vi "CheckStatus_Power_HeaterAlarm.vi"(8 "error in (no error)":errorcluster, 10 "RelayKeyStatus":bool, 11 "DAQmxTaksContainer_General in":refnum<class "DAQmxTaksContainer_General.lvclass">) -> (0 "error out":errorcluster, 1 "PowerStatus":bool, 2 "PowerStatusChanged":bool, 3 "DAQmxTaksContainer_General out":refnum<class "DAQmxTaksContainer_General.lvclass">, 4 "DAQmxTaskAICurrent en sortie":refnum<class "DAQmxTaskAICurrent_General.lvclass">, 5 "HeaterAlarmStatus":bool, 7 "HeaterAlarmStatusChanged":bool)   [LabVIEW 2018, in "DAQmxTaksContainer_General.lvclass"]
uses:
  DAQmxTaksContainer_General.lvclass
  DAQmxTaskAICurrent_General/DAQmxTaskAICurrent_General.lvclass
  DAQmxTaksContainer_General.lvclass/DAQmxTaksContainer_General.ctl
  DAQmxTaskAICurrent_General/DAQmxTaskAICurrent_General.lvclass/DAQmxTaskAICurrent_General.ctl
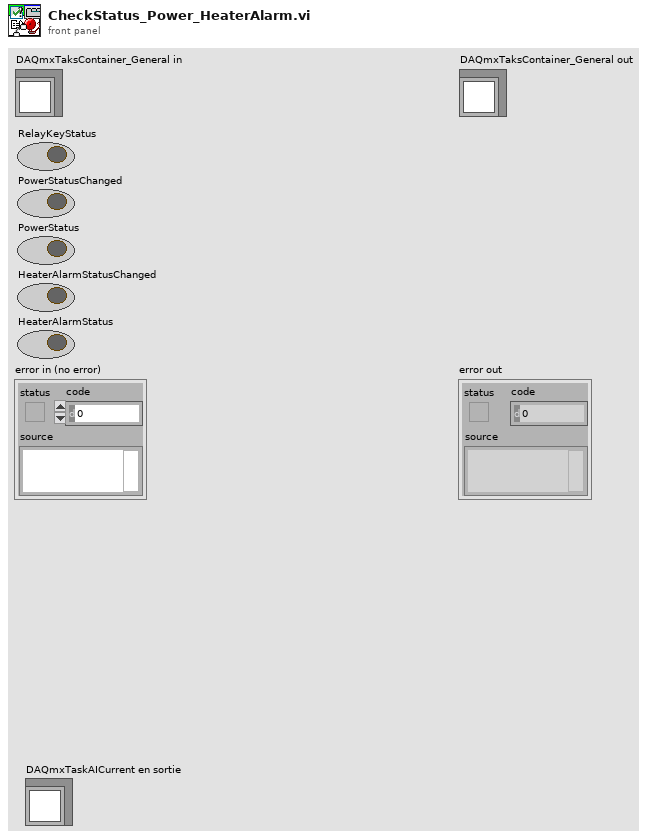
[diagram p1: front panel]
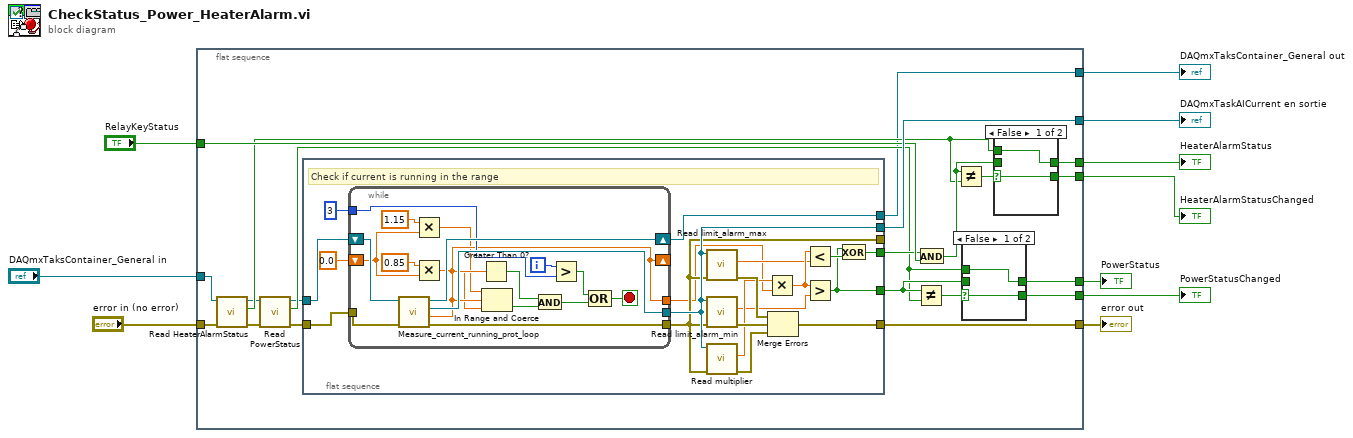
[diagram p0: block diagram]
diagram:
  n1 = flat-sequence {
    tunnel: "DAQmxTaksContainer_General in" -> [w17]
    tunnel: "error in (no error)" -> [w15]
    tunnel: [w31] -> w1
    tunnel: [w30] -> w5
    tunnel: "RelayKeyStatus" -> [w29]
    tunnel: [w25] -> w7
    tunnel: [w24] -> w8
    tunnel: [w22] -> w9
    tunnel: [w20] -> w10
    tunnel: [w11] -> w2
    frame #0 {
      n2 = call "Read HeaterAlarmStatus.vi"("error in (no error)"=w15, "DAQmxTaksContainer_General in"=w17) -> ("error out"=w14:errorcluster, "HeaterAlarmStatus"=w19:bool, "DAQmxTaksContainer_General out"=w16:refnum<class "DAQmxTaksContainer_General.lvclass">)  [unwired: 7 in]
      n3 = call "Read PowerStatus.vi"("error in (no error)"=w14, "DAQmxTaksContainer_General in"=w16) -> ("error out"=w13:errorcluster, "PowerStatus"=w18:bool, "DAQmxTaksContainer_General out"=w12:refnum<class "DAQmxTaksContainer_General.lvclass">)  [unwired: 7 in]
      n4 = flat-sequence {
        tunnel: [w44] -> w31
        tunnel: [w43] -> w30
        tunnel: [w42] -> _
        tunnel: [w39] -> w28
        tunnel: [w38] -> w26
        tunnel: w13 -> [w37]
        tunnel: w12 -> [w36]
        tunnel: [w35] -> w11
        frame #0 {
          # "Check if current is running in the range"
          n5 = while {
            tunnel: [w68] -> w43
            tunnel: [w56] -> w34
            shift-right: [w64] -> w35
            shift-left: w36 -> [w65]
            tunnel: w37 -> [w66]
            tunnel: [w67] -> w42
            shift-right: [w56] -> _
            shift-left: 0.0 ("value") -> [w53]
            tunnel: 3 -> [w62]
            i -> [w63]
            stop <- w60 stop-if-true
            n6 = call "Measure_current_running_prot_loop.vi"("error in (no error)"=w66, "DAQmxTaksContainer_General in"=w65) -> ("error out"=w67:errorcluster, "value"=w56:dbl, "DAQmxTask en sortie"=w68:refnum<class "DAQmxTaskAICurrent_General.lvclass">, "DAQmxTaksContainer_General out"=w64:refnum<class "DAQmxTaksContainer_General.lvclass">)  [unwired: 6 in]
            n7 = Multiply(x=1.15, y=w53) -> (x*y=w55:dbl)
            n8 = Multiply(x=0.85, y=w53) -> (x*y=w54:dbl)
            n9 = Greater Than 0?(x=w56) -> (x > 0?=w59:bool)
            n10 = In Range and Coerce(upper limit=w55, x=w56, lower limit=w54) -> (In Range?=w57:bool)  [unwired: 1 out]
            n11 = And(x=w59, y=w57) -> (x .and. y?=w58:bool)
            n12 = Greater?(x=w63, y=w62) -> (0:w61:bool)
            n13 = Compound Arithmetic op=OR(w61, w58) -> (w60:bool)
          }
          n14 = call "Read limit_alarm_max.vi"("error in (no error)"=w42, "DAQmxTaskAICurrent_General in"=w43) -> ("error out"=w46:errorcluster, "limit_alarm_max"=w40:dbl)  [unwired: 7 in, 1 out]
          n15 = call "Read limit_alarm_min.vi"("error in (no error)"=w42, "DAQmxTaskAICurrent_General in"=w43) -> ("error out"=w47:errorcluster, "limit_alarm_min"=w41:dbl)  [unwired: 7 in, 1 out]
          n16 = call "Read multiplier.vi"("error in (no error)"=w42, "DAQmxTaskAICurrent_General in"=w43) -> ("error out"=w48:errorcluster, "multiplier"=w45:dbl)  [unwired: 7 in, 1 out]
          n17 = Multiply(x=w45, y=w34) -> (x*y=w49:dbl)
          n18 = Merge Errors(w46, w47, w48) -> (w44:errorcluster)
          n19 = Less?(x=w49, y=w40) -> (x < y?=w50:bool)
          n20 = Greater?(x=w49, y=w41) -> (0:w38:bool)
          n21 = Exclusive Or(1:w50, 2:w38) -> (0:w39:bool)
        }
      }
      n22 = Not Equal?(x=w26, y=w18) -> (x != y?=w27:bool)
      n23 = And(x=w28, y=w29) -> (x .and. y?=w21:bool)
      n24 = Not Equal?(x=w21, y=w19) -> (x != y?=w23:bool)
      n25 = case shown="False" w27 {
        selector: w27 -> [w74 w75]
        tunnel: [w74 w75] -> w25
        tunnel: w26 -> [_ w76]
        tunnel: [w73 w76] -> w24
        tunnel: w18 -> [w73 _]
        frame False {
        }
        frame True {
        }
      }
      n26 = case shown="False" w23 {
        selector: w23 -> [w70 w72]
        tunnel: [w70 w72] -> w22
        tunnel: [w69 w71] -> w20
        tunnel: w21 -> [_ w71]
        tunnel: w19 -> [w69 _]
        frame False {
        }
        frame True {
        }
      }
    }
  }
  "error out" <- w1
  "DAQmxTaksContainer_General out" <- w2
  "HeaterAlarmStatus" <- w10
  "HeaterAlarmStatusChanged" <- w9
  "PowerStatus" <- w8
  "PowerStatusChanged" <- w7
  "DAQmxTaskAICurrent en sortie" <- w5
